vi "TCP_setup.vi"(8 "address":string, 10 "remote port or service name":u16=7776) -> (0 "error out":errorcluster, 3 "TCP Network Connection out":refnum<k5>)   [LabVIEW 2019]
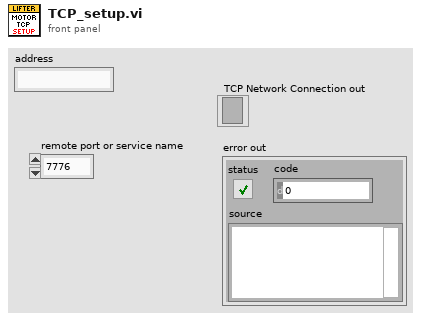
[diagram p1: front panel]
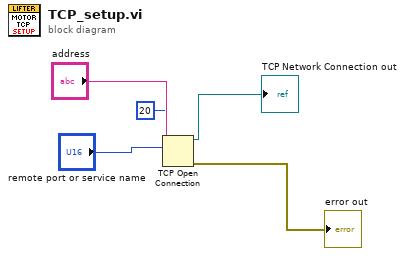
[diagram p0: block diagram]
diagram:
  n1 = TCP Open Connection(address="address", remote port or service name="remote port or service name", timeout ms (60000)=20) -> (connection ID=→"TCP Network Connection out":refnum<k5>, error out=→"error out":errorcluster)  [unwired: 2 in]
